vi "Create Database.vi"(8 "error in (no error)":errorcluster caption="错误输入（无错误）") -> (0 "error out":errorcluster caption="错误输出")   [LabVIEW 2018]
uses:
  <vilib>/Utility/NIReport.llb/Report Type.ctl
  <vilib>/drjdpowell/SQLite Library/SQL Connection/Connection.lvclass
  <vilib>/drjdpowell/SQLite Library/SQL Connection/Open (path).vi
  <vilib>/drjdpowell/SQLite Library/SQL Connection/Open (string).vi
  <vilib>/addons/_office/excel.llb/Excel Get Data ([str]).vi
  <vilib>/AdvancedString/Path To Command Line String.vi
  <vilib>/drjdpowell/SQLite Library/SQL Connection/Execute SQL (No results).vi
  <vilib>/Utility/NIReport.llb/NI_report.lvclass
  <vilib>/Utility/NIReport.llb/Excel/NI_Excel.lvclass
  <vilib>/Utility/NIReport.llb/NI_ReportGenerationCore.lvlib
  <vilib>/addons/_office/NI_ReportGenerationToolkit.lvlib
  <vilib>/drjdpowell/SQLite Library/SQLite.lvlib
panel:
  out "x-y":u32
  out "连接的字符串":string
  out "数组":string[][](array[string])
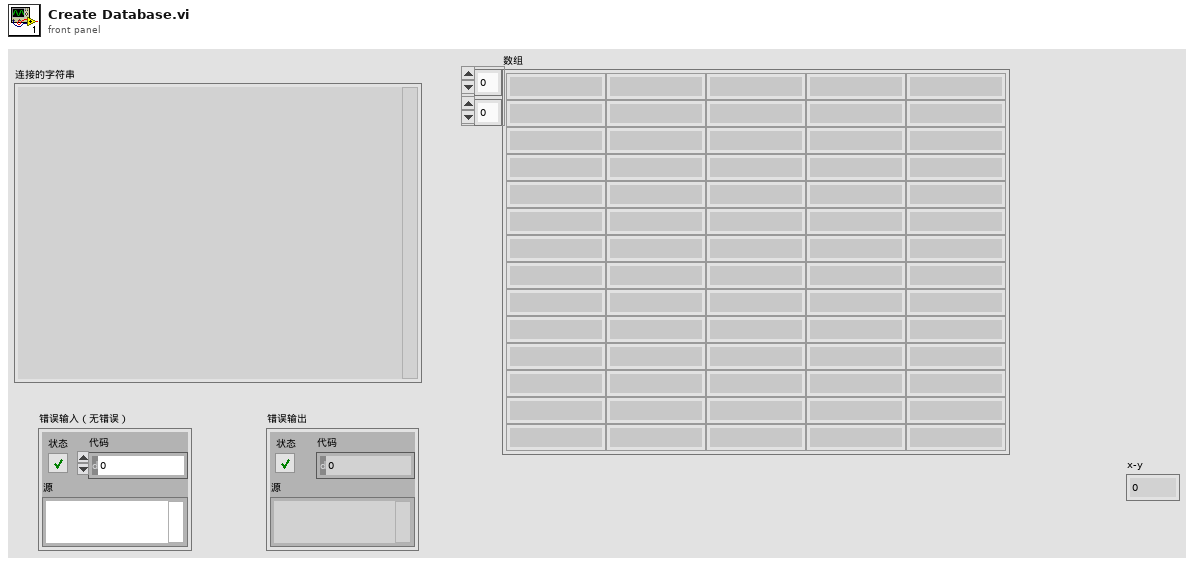
[diagram p1: front panel]
types:
  T1 = enum16{"maximized", "minimized", "normal", "no change"}
  T2 = typedef "NI_ReportGenerationCore.lvlib/Report Type.ctl" = enum16{"HTML", "Word", "Excel"}
  T3 = enum16{"New or existing", "Existing", "Read only"}
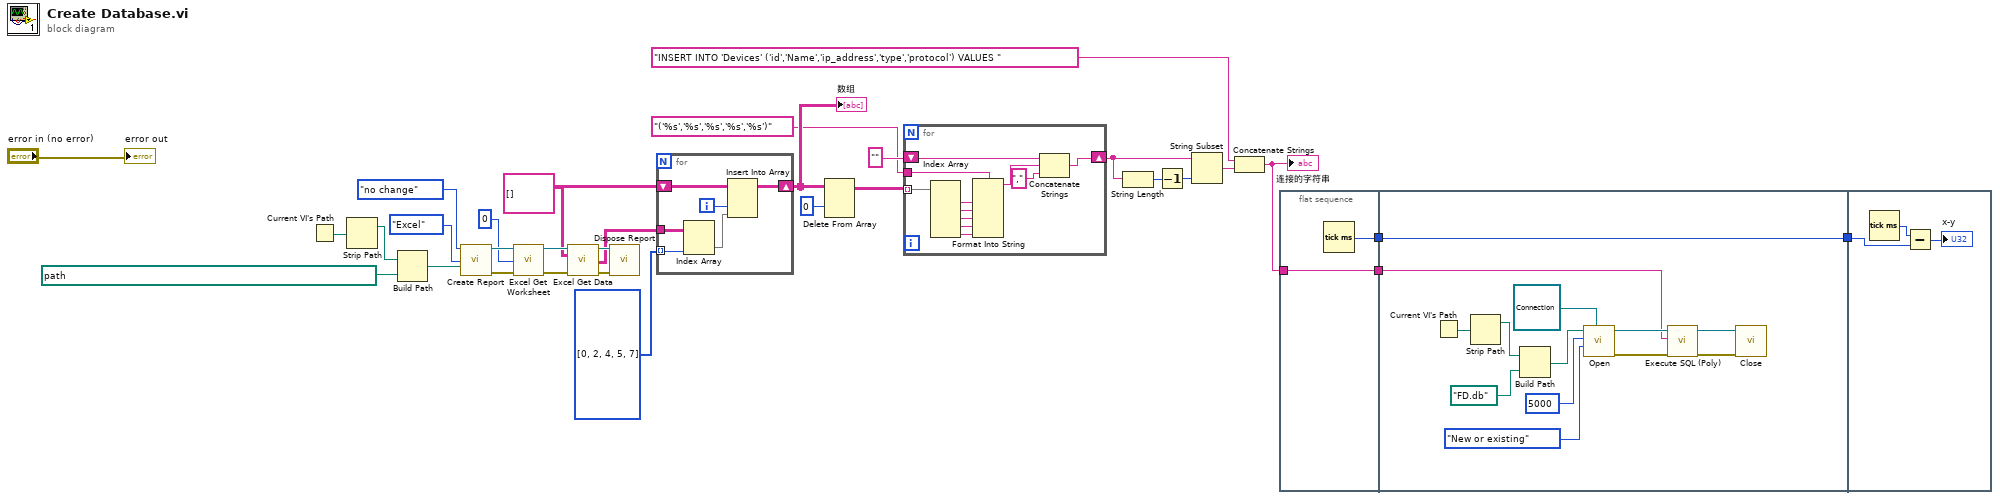
[diagram p0: block diagram]
diagram:
  w16 = string[][] []
  n1 = Current VI's Path() -> (path=w21:path)
  n2 = Strip Path(path=w21) -> (stripped path=w20:path)  [unwired: 1 out]
  n3 = Build Path(base path=w20, name or relative path=path "../Document/7.交直流配电板及其配电开关IP地址需求表.xlsx" ("template (empty)")) -> (appended path=w19:path)
  n4 = call <vilib>:"Create Report.vi"("window state (normal)"=T1."no change", "report type"=Report_Type."Excel", "template (empty)"=w19) -> ("report out"=w30:refnum<class "NI_report.lvclass">, "error out"=w28:errorcluster)  [unwired: 11 in]
  n5 = call <vilib>:"Excel Get Worksheet.vi"("report in"=w30, "worksheet index (0)"=0, "error in (no error)"=w28) -> ("report out"=w25:refnum<class "NI_report.lvclass">, "error out"=w23:errorcluster)  [unwired: 11 in]
  n6 = call-poly <vilib>:"Excel Get Data.vi"("report in"=w25, "data type"=w16, "error in (no error)"=w23) -> ("report out"=w24:refnum<class "NI_report.lvclass">, "data"=w17:string[][], "error out"=w22:errorcluster)  [unwired: 10 in]
  n7 = call-dynamic "Dispose Report.vi"("report in"=w24, "error in (no error)"=w22) -> ()  [unwired: 13 in, 1 out]
  n8 = for {
    shift-right: [w36] -> w13
    shift-left: w16 -> [w37]
    tunnel: i32[] [0, 2, 4, 5, 7] ("索引") -> [w32] mode=indexing
    tunnel: w17 -> [w35]
    i -> [w33]
    n9 = Index Array(array=w35, index (col)=w32) -> (element=w34:string[])  [unwired: 1 in]
    n10 = Insert Into Array(array=w37, index (col)=w33, new element=w34) -> (w36:string[][])  [unwired: 1 in]
  }
  "数组" <- w13
  n11 = Delete From Array(array=w13, index (row)=0 ("索引 (行)")) -> (array with subset deleted=w11:string[][])  [unwired: 2 in, 1 out]
  n12 = for {
    tunnel: w11 -> [w48] mode=indexing
    tunnel: "('%s','%s','%s','%s','%s')" -> [w42]
    shift-right: [w41] -> w6
    shift-left: "" -> [w40]
    n13 = Index Array(array=w48) -> (element #1=w47:string, element #2=w46:string, element #3=w45:string, element #4=w44:string, element #5=w43:string)  [unwired: 5 in]
    n14 = Format Into String(format string=w42, w47, w46, w45, w44, w43) -> (resulting string=w39:string)  [unwired: 2 in, 1 out]
    n15 = Concatenate Strings(w40, w39, ",") -> (w41:string)
  }
  n16 = String Length(string=w6) -> (length=w9:i32)
  n17 = Decrement(x=w9) -> (x-1=w8:i32)
  n18 = String Subset(string=w6, length (rest)=w8) -> (substring=w7:string)  [unwired: 1 in]
  n19 = Concatenate Strings("INSERT INTO 'Devices' ('id','Name','ip_address','type','protocol') VALUES ", w7) -> (w1:string)
  "连接的字符串" <- w1
  n20 = flat-sequence {
    tunnel: [w50] -> w4
    tunnel: [w49] -> w3
    tunnel: w1 -> [w49]
    tunnel: w4 -> [w63]
    tunnel: [w63] -> w2
    tunnel: w3 -> [w53]
    tunnel: w2 -> [w65]
    frame #0 {
      n21 = Tick Count (ms)() -> (millisecond timer value=w50:u32)
    }
    frame #1 {
      n22 = Current VI's Path() -> (path=w59:path)
      n23 = Strip Path(path=w59) -> (stripped path=w58:path)  [unwired: 1 out]
      n24 = Build Path(base path=w58, name or relative path=path "FD.db" ("template (empty)")) -> (appended path=w57:path)
      n25 = call-poly <vilib>:"Open.vi"("SQLite Connection type"=refnum<class "Connection.lvclass"> refnum, "File Option"=T3."New or existing", "busy timeout (ms)"=5000, "db file"=w57) -> ("error out"=w51:errorcluster, "SQLite Connection"=w55:refnum<class "Connection.lvclass">)  [unwired: 6 in]
      n26 = call-poly <vilib>:"Execute SQL (Poly).vi"("error in (no error)"=w51, "SQL"=w53, "SQLite Connection in"=w55) -> ("error out"=w52:errorcluster, "SQLite Connection"=w54:refnum<class "Connection.lvclass">)  [unwired: 7 in]
      n27 = call-dynamic "Close.vi"("error in (no error)"=w52, "SQLite Connection in"=w54) -> ()  [unwired: 9 in, 1 out]
    }
    frame #2 {
      n28 = Tick Count (ms)() -> (millisecond timer value=w66:u32)
      n29 = Subtract(x=w66, y=w65) -> (x-y=→"x-y":u32)
    }
  }
  "error out" <- "error in (no error)"
